vi "Dequeue_Data.vi"(6 "error in (no error)":errorcluster, 9 "Ref in":T2 {"TS Parameter"."FCA" format="%01d"; "TS Parameter"."Target" min=1 max=100000; "TS Parameter"."PokaYoke" min=0 max=1}) -> (0 "error out":errorcluster, 3 "Ref Out":T2 {"TS Parameter"."FCA" format="%01d"; "TS Parameter"."Target" min=1 max=100000; "TS Parameter"."PokaYoke" min=0 max=1}, 4 "TS Parameter":T1={"ProfitCenterCode"="", "LineCode"="", "WorkOrderNumber"="", "Model"="", "Model_with_Prefix"="", "VendorCode"="", "SetParameterDateCode"="", "PokaYoke"=0, "Target"=1, "Live_DateCode"="", "CustomerPartNumber"="", "Hand"="", "sBarcode"=FALSE, "FCA"=0, "Ent_Stamp"=timestamp(0 s since 1904-01-01), "STS_CD"=0.0} {"FCA" format="%01d"; "Target" min=1 max=100000; "PokaYoke" min=0 max=1}, 5 "Data Change":bool)   [LabVIEW 2020]
uses:
  Controls/TD SQL.ctl
  <vilib>/addons/database/Connection.llb/Conn ObjectReference.ctl
  Controls/WIP_State.ctl
  Controls/TS_Parameter.ctl
  <vilib>/addons/database/NI_Database_API.lvlib
panel:
  out "queue name":string
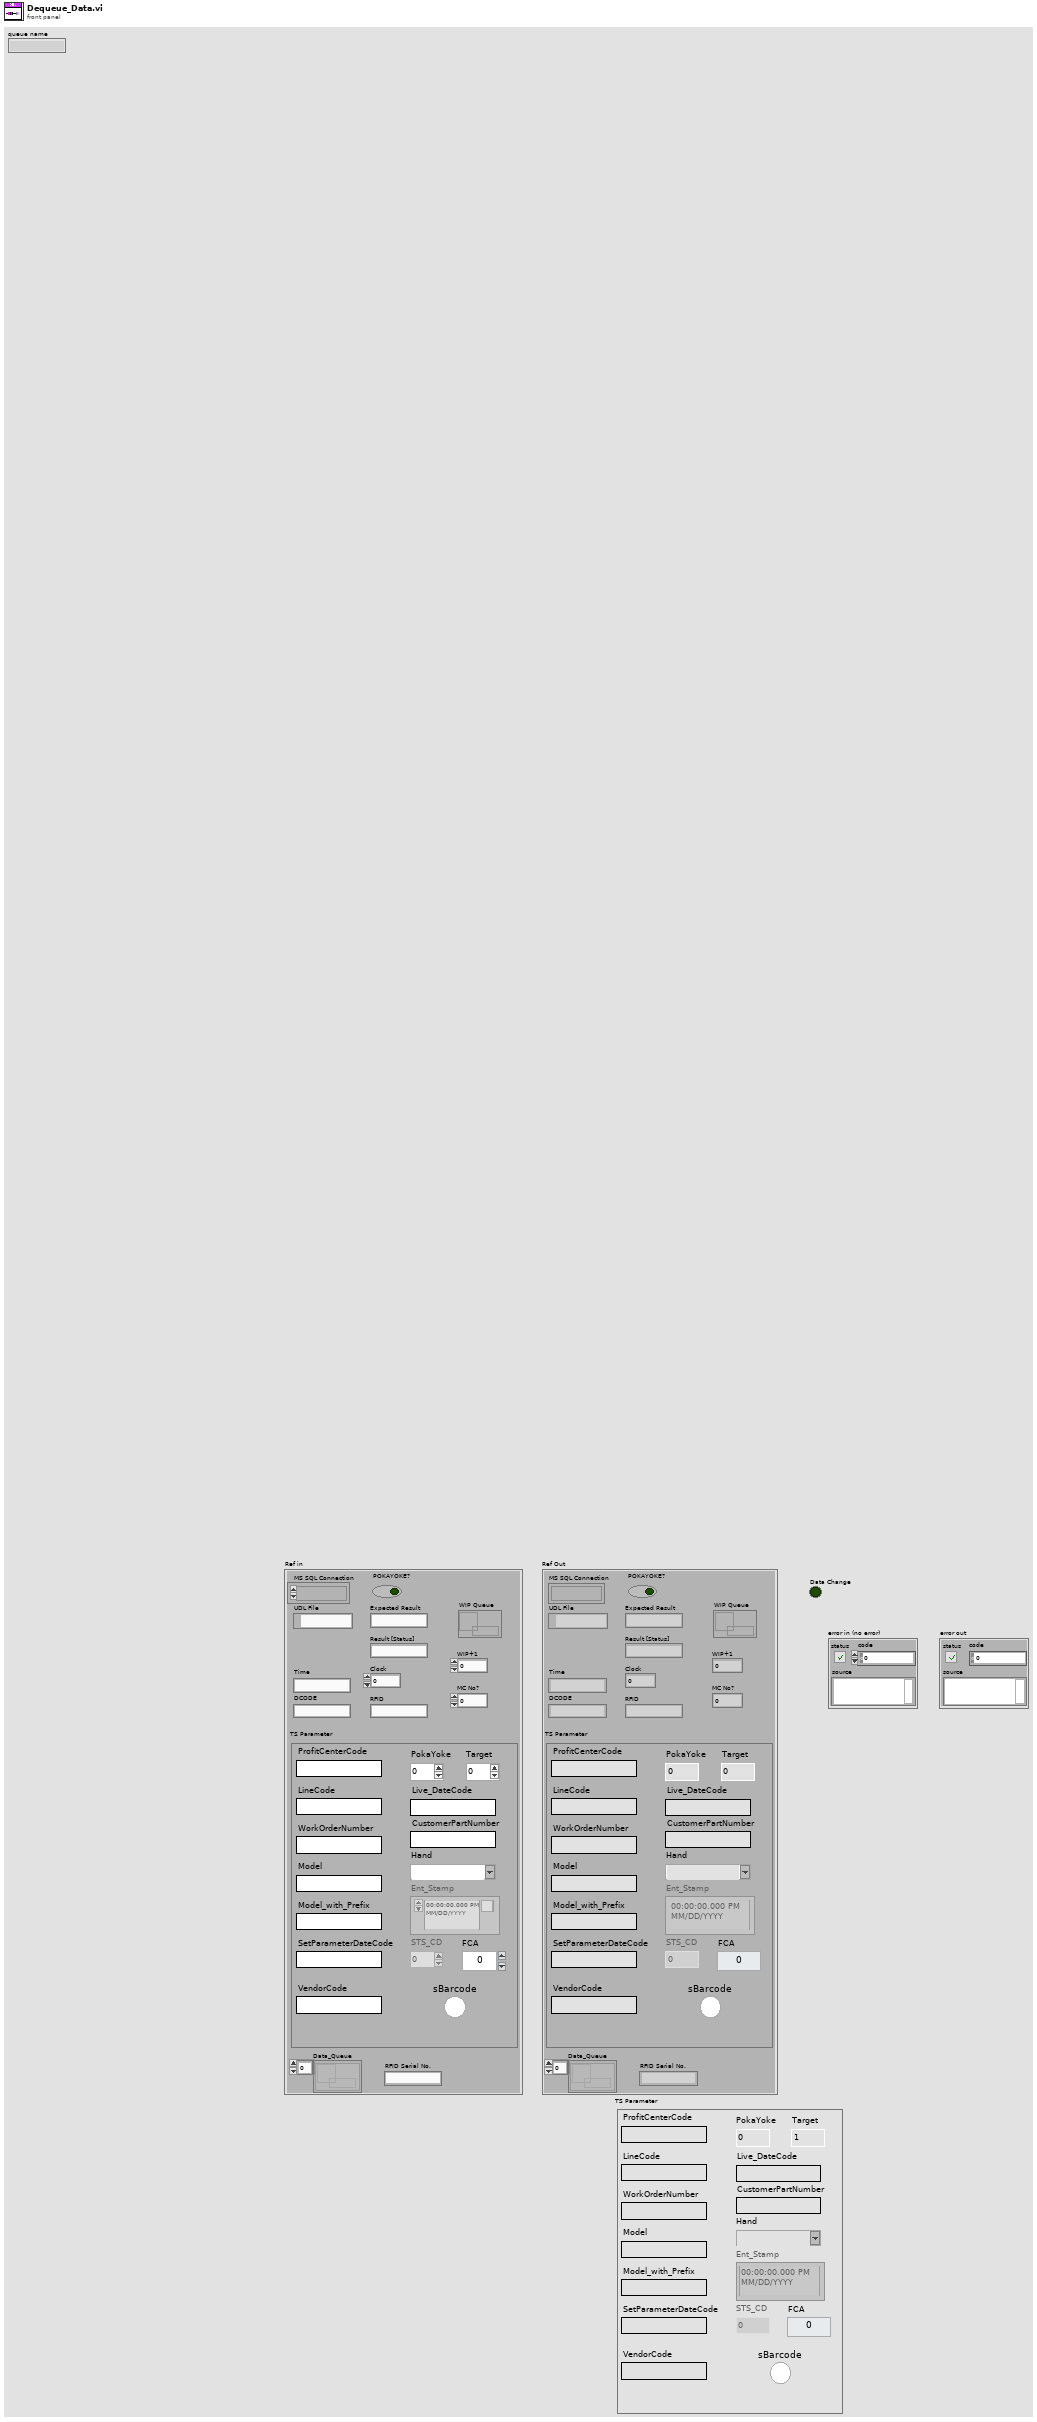
[diagram p1: front panel]
types:
  T1 = typedef "TS_Parameter.ctl" = cluster{"ProfitCenterCode":string, "LineCode":string, "WorkOrderNumber":string, "Model":string, "Model_with_Prefix":string, "VendorCode":string, "SetParameterDateCode":string, "PokaYoke":i32, "Target":i32, "Live_DateCode":string, "CustomerPartNumber":string, "Hand":string, "sBarcode":bool, "FCA":i32, "Ent_Stamp":timestamp, "STS_CD":dbl}
  T2 = typedef "TD SQL.ctl" = cluster{"MS SQL Connection":T3, "UDL File":path, "Time":string, "DCODE":string, "WIP+1":i64, "MC No?":i32, "POKAYOKE?":bool, "Expected Result":string, "Result [Status]":string, "Clock":dbl, "RFID":string, "WIP Queue":refnum<queue>, "TS Parameter":T1, "Data_Queue":refnum<queue>[], "RFID Serial No.":string}
  T3 = typedef "NI_Database_API.lvlib/Conn ObjectReference.ctl" = refnum<k1>
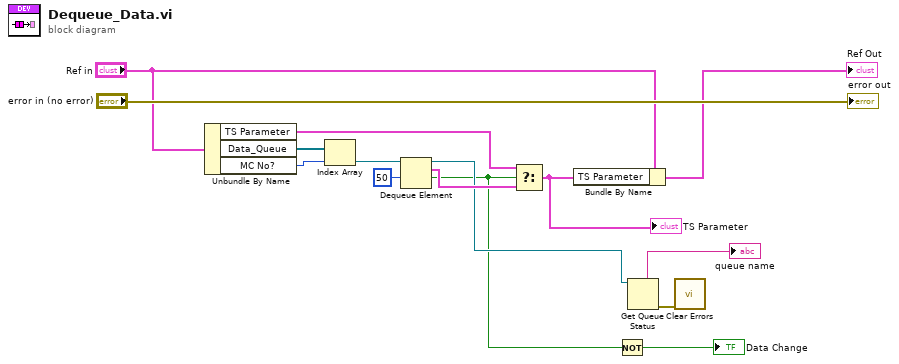
[diagram p0: block diagram]
diagram:
  n1 = Unbundle By Name("Ref in") -> ("TS Parameter"=w10:T1, "Data_Queue"=w9:refnum<queue>[], "MC No?"=w8:i32)
  n2 = Index Array(array=w9, index=w8) -> (element=w14:refnum<queue>)
  n3 = Dequeue Element(queue=w14, timeout in ms (-1)=50) -> (queue out=w5:refnum<queue>, element=w12:T1, timed out?=w3:bool)  [unwired: 1 in, 1 out]
  n4 = Select(t=w10, s=w3, f=w12) -> (s? t:f=w1:T1)
  "TS Parameter" <- w1
  n5 = Bundle By Name(cluster="Ref in", "TS Parameter"=w1) -> (→"Ref Out":T2)
  n6 = Not(x=w3) -> (.not. x?=→"Data Change":bool)
  n7 = Get Queue Status(queue=w5) -> (queue name=→"queue name":string, error out=w7:errorcluster)  [unwired: 2 in, 6 out]
  n8 = call <vilib>:"Clear Errors.vi"("error in (no error)"=w7) -> ()  [unwired: 5 in, 2 out]
  "error out" <- "error in (no error)"
